vi "test.vi"() -> ()   [LabVIEW 2026]
uses:
  target/debug/labview_test_library.dll
  <vilib>/Utility/Data Type/NI_Data Type.lvlib
panel:
  out "result 4":string
  out "return type 4":i32
  out "x = y? 3":bool
  out "result 3":i8
  out "return type 3":i32
  out "x = y? 2":bool
  out "x = y?":bool
  out "result 2":dbl format="%#_6f"
  out "return type 2":i32
  out "variant":variant
  out "error out":errorcluster
  out "result":i32
  out "return type":i32
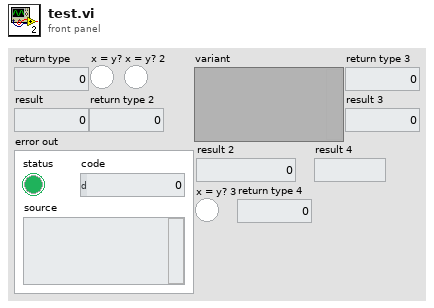
[diagram p1: front panel]
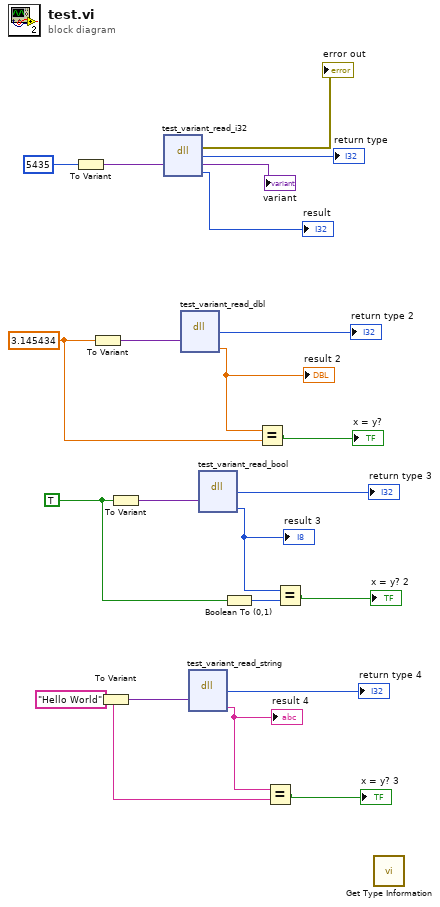
[diagram p0: block diagram]
diagram:
  w5 = "Hello World"
  w8 = TRUE
  w13 = 3.145434
  n1 = To Variant(anything=5435) -> (Variant=w19:variant)
  n2 = To Variant(anything=w13) -> (Variant=w16:variant)
  n3 = To Variant(anything=w5) -> (Variant=w4:variant)
  n4 = To Variant(anything=w8) -> (Variant=w9:variant)
  n5 = dll-call lib="C:/Git/Rust-LabVIEW-Interop/target/debug/labview_test_library.dll" fn="test_variant_read_i32"("variant"=w19) -> (error out=→"error out":errorcluster, "return type"=→"return type":i32, "variant"=→"variant":variant, "result"=→"result":i32)  [unwired: 4 in, 1 out]
  n6 = dll-call lib="C:/Git/Rust-LabVIEW-Interop/target/debug/labview_test_library.dll" fn="test_variant_read_dbl"("variant"=w16) -> ("return type"=→"return type 2":i32, "result"=w14:dbl)  [unwired: 5 in, 2 out]
  "result 2" <- w14
  n7 = dll-call lib="C:/Git/Rust-LabVIEW-Interop/target/debug/labview_test_library.dll" fn="test_variant_read_string"("variant"=w4) -> ("return type"=→"return type 4":i32, "result"=w1:string)  [unwired: 5 in, 2 out]
  "result 4" <- w1
  n8 = dll-call lib="C:/Git/Rust-LabVIEW-Interop/target/debug/labview_test_library.dll" fn="test_variant_read_bool"("variant"=w9) -> ("return type"=→"return type 3":i32, "result"=w6:i8)  [unwired: 5 in, 2 out]
  "result 3" <- w6
  n9 = Boolean To (0,1)(Boolean=w8) -> (0, 1=w7:i16)
  n10 = Equal?(x=w14, y=w13) -> (x = y?=→"x = y?":bool)
  n11 = Equal?(x=w1, y=w5) -> (x = y?=→"x = y? 3":bool)
  n12 = Equal?(x=w6, y=w7) -> (x = y?=→"x = y? 2":bool)
  n13 = call <vilib>:"Get Type Information.vi"() -> ()  [unwired: 7 in, 5 out]
